vi "創造圖片(2D).vi"(0 "ImageNameArray":string[](array[string])=["Source"], 5 "影像數量":i32=1, 11 "error In":errorcluster) -> (4 "Image2DArray":T1[][](array[typedef]), 6 "ImageNameNumber":i32, 10 "ImageOutNameArray":string[](array[string]), 15 "error out":errorcluster)   [LabVIEW 2015]
uses:
  <vilib>/vision/Image Controls.llb/IMAQ Image.ctl
  Image action.ctl
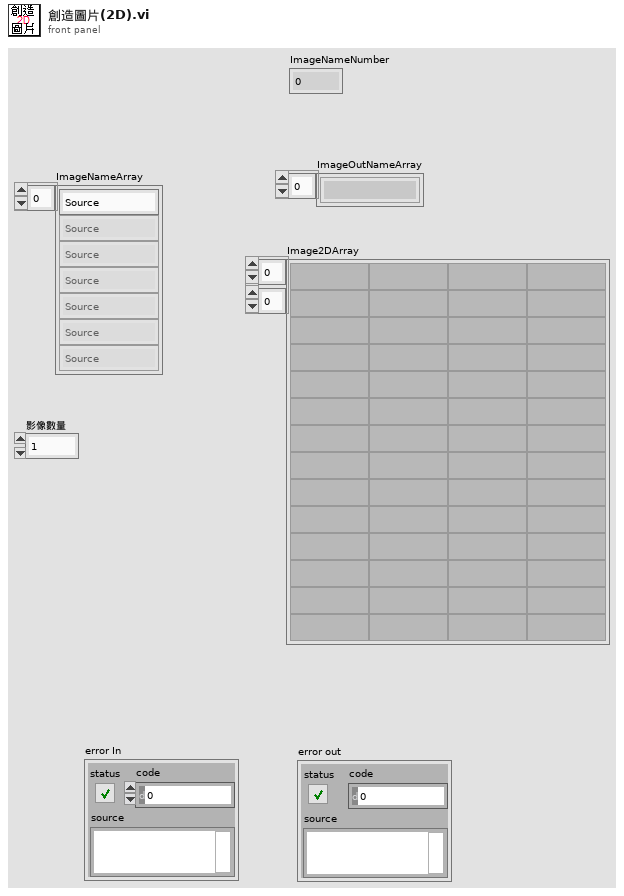
[diagram p1: front panel]
types:
  T1 = typedef "IMAQ Image.ctl" = refnum<image>
  T2 = typedef "Image action.ctl" = enum16{"初始化", "創造記憶體", "寫入圖片", "讀取圖片", "刪除圖片", "等待"}
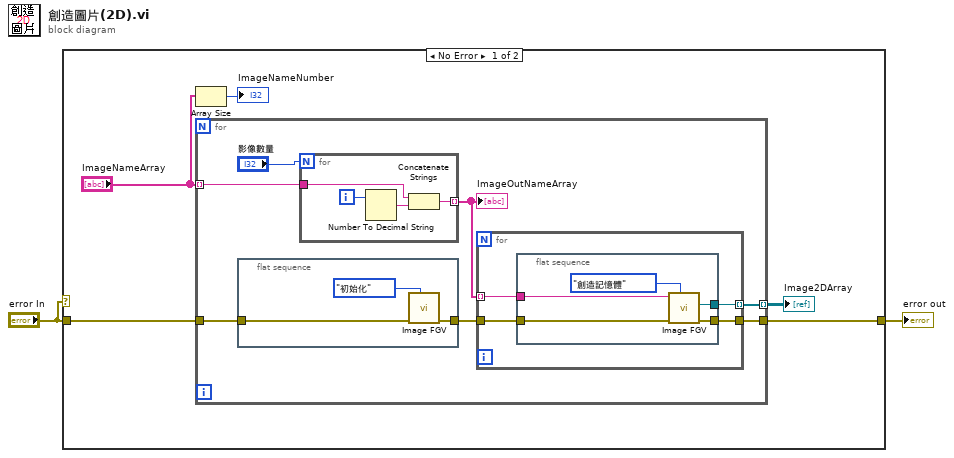
[diagram p0: block diagram]
diagram:
  n1 = case shown="No Error" "error In" {
    tunnel: [w5 w31] -> w2
    tunnel: "error In" -> [w6 w31]
    frame No Error {
      n2 = Array Size(array="ImageNameArray") -> (size(s)=→"ImageNameNumber":i32)
      n3 = for {
        tunnel: "ImageNameArray" -> [w13] mode=indexing
        tunnel: [w9] -> w7 mode=indexing
        tunnel: w6 -> [w10]
        tunnel: [w8] -> w5
        n4 = flat-sequence {
          tunnel: [w29] -> w14
          tunnel: w10 -> [w28]
          frame #0 {
            n5 = call "Image FGV.vi"("Image action"=Image_action."初始化", "error in (no error)"=w28) -> ("error out"=w29:errorcluster)  [unwired: 8 in, 1 out]
          }
        }
        n6 = for {
          N: "影像數量" -> [_]
          tunnel: w13 -> [w17]
          tunnel: [w15] -> w11 mode=indexing
          i -> [w18]
          n7 = Number To Decimal String(number=w18) -> (decimal integer string=w16:string)  [unwired: 1 in]
          n8 = Concatenate Strings(w17, w16) -> (w15:string)
        }
        "ImageOutNameArray" <- w11
        n9 = for {
          tunnel: w14 -> [w22]
          tunnel: w11 -> [w21] mode=indexing
          tunnel: [w20] -> w8
          tunnel: [w19] -> w9 mode=indexing
          n10 = flat-sequence {
            tunnel: w22 -> [w26]
            tunnel: w21 -> [w25]
            tunnel: [w24] -> w20
            tunnel: [w23] -> w19
            frame #0 {
              n11 = call "Image FGV.vi"("Image action"=Image_action."創造記憶體", "error in (no error)"=w26, "圖片名稱"=w25) -> ("error out"=w24:errorcluster, "Image Out"=w23:T1)  [unwired: 7 in]
            }
          }
        }
      }
      "Image2DArray" <- w7
    }
    frame Error {
    }
  }
  "error out" <- w2
